vi "Message for Adding Model.vi"(7 "eHS Core Index":T1, 8 "Error In":errorcluster, 10 "Number of Loaded Models":i32, 11 "Model File Name":string) -> (0 "Error Out":errorcluster, 3 "Message":string)   [LabVIEW 2017]
uses:
  <vilib>/OPAL-RT/eHS Toolkit/eHS Matrix Generation/_Controls/eHS Core Index.ctl
  <vilib>/OPAL-RT/eHS Toolkit/eHS Matrix Generation/eHS Matrix Generation.lvlib
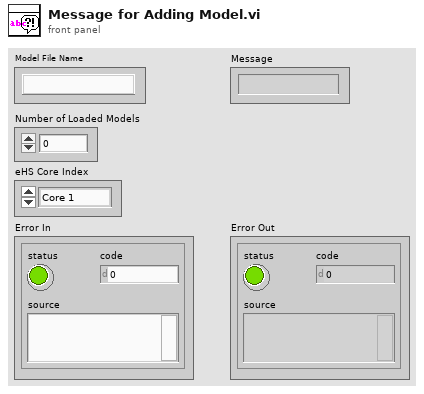
[diagram p1: front panel]
types:
  T1 = typedef "OPAL-RT eHS.lvlib/eHS Matrix Generation.lvlib/eHS Core Index.ctl" = enum16{"Core 1", "Core 2", "Core 3", "Core 4", "Core 5", "Core 6", "Core 7", "Core 8", "Core 9", "Core 10"}
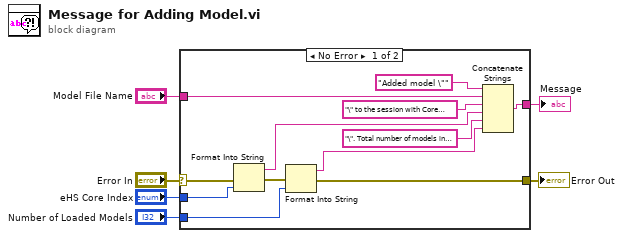
[diagram p0: block diagram]
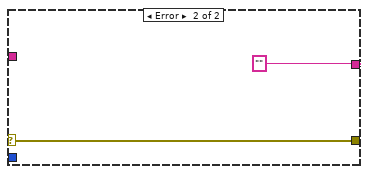
[diagram p2: hidden frame]
diagram:
  n1 = case shown="No Error" "Error In" {
    selector: "Error In" -> [w11 w20]
    tunnel: [w9 w20] -> w5
    tunnel: "Model File Name" -> [w7 _]
    tunnel: [w16 ""] -> w3
    tunnel: "eHS Core Index" -> [w15 _]
    tunnel: "Number of Loaded Models" -> [w12 _]
    frame No Error {
      n2 = Format Into String(error in=w11, w15) -> (resulting string=w8:string, error out=w10:errorcluster)  [unwired: 2 in]
      n3 = Format Into String(error in=w10, w12) -> (resulting string=w13:string, error out=w9:errorcluster)  [unwired: 2 in]
      n4 = Concatenate Strings("Added model \"" ("string"), w7, "\" to the session with Core Index \"" ("string"), w8, "\". Total number of models in session is: " ("string"), w13) -> (w16:string)
    }
    frame Error {
    }
  }
  "Message" <- w3
  "Error Out" <- w5
